vi "Get Properties.vi"(0 "VI Name":string caption="VI Name (\"\")", 5 "AppInst":refnum<vi>, 9 "Scope (0:All)":enum16{"All", "Dynamic"}(ring), 11 "error in":errorcluster) -> (2 "Modifications:VI Modifications Bitset":u64, 3 "File Name Out":string, 4 "Full Name Out":string, 6 "Column Labels":string[](array[string])=["VI Name", "State", "Reentrant", "Reentrancy Type", "FP Behavior", "Code Size", "Data Size", "VI Path"], 8 "Path":path, 10 "Column Data Type":enum16{"String", "Numeric"}[](array[ring]), 12 "ColumnOffsets (Dyn)":i32[](array[numeric])=[1, 1, 1, 5], 13 "VI Properties (Dyn)":string[](array[string]), 14 "VI Properties (All)":string[](array[string]), 15 "error out":errorcluster)   [LabVIEW 2013, in "LVTM.lvlib"]
doc: "Gets the properties at run time of each VI in memory. Set Scope=All to get all properties, set Scope=Dynamic to get only the properties that might change while executing. The later mode will be faster."
uses:
  LVTM.lvlib
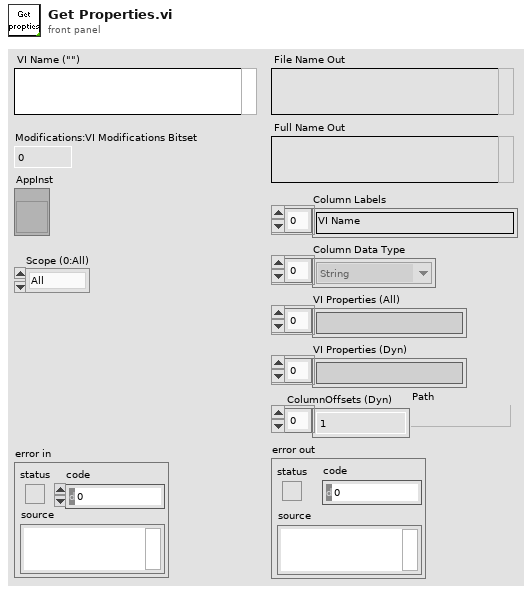
[diagram p1: front panel]
types:
  T1 = enum32{"Bad", "Idle", "Run top level", "Running"}
  T2 = enum16{"Share clones between instances", "Preallocate clone for each instance"}
  T3 = enum32{"Invalid", "Default", "Floating", "Floating/Auto-Hide", "Modal"}
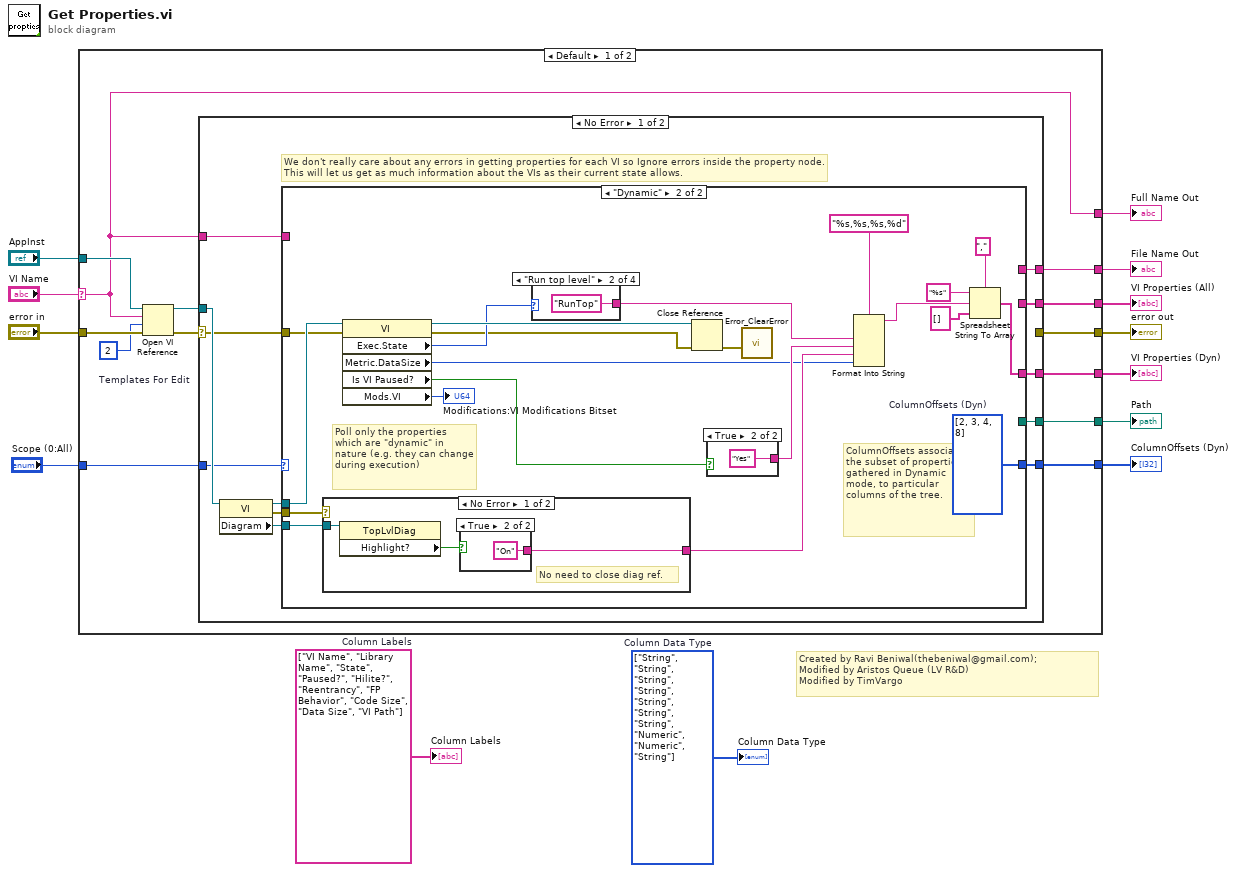
[diagram p0: block diagram]
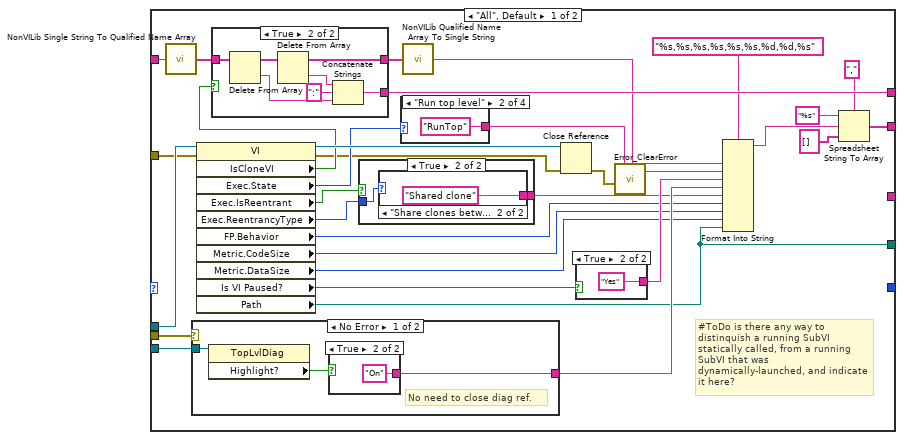
[diagram p2: hidden frame]
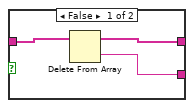
[diagram p3: hidden frame]
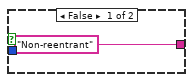
[diagram p4: hidden frame]
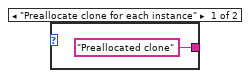
[diagram p5: hidden frame]
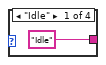
[diagram p6: hidden frame]
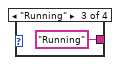
[diagram p7: hidden frame]
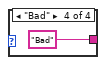
[diagram p8: hidden frame]
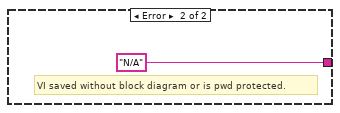
[diagram p10: hidden frame]
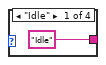
[diagram p12: hidden frame]
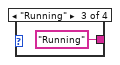
[diagram p13: hidden frame]
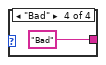
[diagram p14: hidden frame]
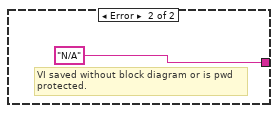
[diagram p16: hidden frame]
diagram:
  w9 = enum16{"String", "Numeric"}[] [enum."String", enum."String", enum."String", enum."String", enum."String", enum."String", enum."String", enum."Numeric", enum."Numeric", enum."String"] items=["String", "Numeric"]  # Column Data Type
  w12 = string[] ["VI Name", "Library Name", "State", "Paused?", "Hilite?", "Reentrancy", "FP Behavior", "Code Size", "Data Size", "VI Path"]  # Column Labels
  # "Created by Ravi Beniwal(thebeniwal@gmail.com);\nModified by Aristos Queue (LV R&D)\nModified by TimVargo"
  n1 = case shown="Default" "VI Name" {
    selector: "VI Name" -> [w20 w128]
    tunnel: [w26 _] -> w13
    tunnel: "error in" -> [w25 w127]
    tunnel: [w20 w128] -> w10
    tunnel: [w22 _] -> w8
    tunnel: "AppInst" -> [w21 _]
    tunnel: [w18 w127] -> w5
    tunnel: "Scope (0:All)" -> [w17 _]
    tunnel: [w16 _] -> w3
    tunnel: [w15 _] -> w2
    tunnel: [w14 _] -> w1
    frame Default {
      w23 = 2  # Templates For Edit
      n2 = Open VI Reference(application reference (local)=w21, vi path=w20, options=w23, error in (no error)=w25) -> (vi reference=w24:refnum<vi>, error out=w19:errorcluster)  [unwired: 2 out]
      n3 = case shown="No Error" w19 {
        selector: w19 -> [w31 w126]
        tunnel: [w38 _] -> w26
        tunnel: w24 -> [w37 _]
        tunnel: [w36 _] -> w22
        tunnel: w20 -> [w35 _]
        tunnel: [_ w126] -> w18
        tunnel: w17 -> [w30 _]
        tunnel: [w29 _] -> w16
        tunnel: [w28 _] -> w15
        tunnel: [w27 _] -> w14
        frame No Error {
          # "We don't really care about any errors in getting properties for each VI so Ignore errors inside the property node.\nThis will let us get as much information about the VIs as their current state allows."
          n4 = property class="VI"(reference=w37) -> (reference out=w33:refnum<vi>, error out=w34:errorcluster, "Diagram"=w32:refnum<vi>)  [unwired: 1 in]
          n5 = case shown="\"Dynamic\"" w30 {
            tunnel: [w69 _] -> w38
            tunnel: [w68 _] -> w36
            tunnel: w35 -> [w67 _]
            tunnel: w34 -> [w56 w108]
            tunnel: w33 -> [w55 w107]
            tunnel: w32 -> [w54 w106]
            tunnel: w31 -> [w43 w100]
            tunnel: [_ w99] -> w29
            tunnel: [_ w98] -> w28
            tunnel: [w39 _] -> w27
            frame "All", Default {
              # "#ToDo is there any way to distinquish a running SubVI statically called, from a running SubVI that was dynamically-launched, and indicate it here?"
              n6 = call "NonVILib Single String To Qualified Name Array.vi"("Fully Qualified String"=w67) -> ("Fully Qualified Array"=w66:string[])
              n7 = case shown="No Error" w56 {
                tunnel: [w89 "N/A"] -> w50
                tunnel: w54 -> [w91 _]
                frame No Error {
                  # "No need to close diag ref."
                  n8 = property class="TopLvlDiag"(reference=w91) -> ("Highlight?"=w90:bool)  [unwired: 1 in, 2 out]
                  n9 = case shown="True" w90 {
                    tunnel: [_ "On"] -> w89
                    frame False {
                    }
                    frame True {
                    }
                  }
                }
                frame Error {
                  # "VI saved without block diagram or is pwd protected."
                }
              }
              n10 = property class="VI"(reference=w55, error in=w43) -> (reference out=w63:refnum<vi>, error out=w42:errorcluster, "IsCloneVI"=w44:bool, "Exec.State"=w53:T1, "Exec.IsReentrant"=w46:bool, "Exec.ReentrancyType"=w40:T2, "FP.Behavior"=w47:T3, "Metric.CodeSize"=w48:u32, "Metric.DataSize"=w49:u32, "Is VI Paused?"=w57:bool, "Path"=w39:path)
              n11 = case shown="True" w44 {
                tunnel: w66 -> [w72 w79]
                tunnel: [w71 w73] -> w68
                tunnel: [w70 w77] -> w65
                frame False {
                  n12 = Delete From Array(array=w72) -> (deleted portion=w71:string, array with subset deleted=w70:string[])  [unwired: 2 in]
                }
                frame True {
                  n13 = Delete From Array(array=w79) -> (deleted portion=w75:string, array with subset deleted=w78:string[])  [unwired: 2 in]
                  n14 = Delete From Array(array=w78) -> (deleted portion=w76:string, array with subset deleted=w77:string[])  [unwired: 2 in]
                  n15 = Concatenate Strings(w76, ":" ("element"), w75) -> (w73:string)
                }
              }
              n16 = case shown="True" w46 {
                tunnel: ["Non-reentrant" w82] -> w45
                tunnel: w40 -> [_ w81]
                frame False {
                }
                frame True {
                  n17 = case shown="\"Share clones between instances\"" w81 {
                    tunnel: ["Preallocated clone" "Shared clone"] -> w82
                    frame "Preallocate clone for each instance" {
                    }
                    frame "Share clones between instances" {
                    }
                  }
                }
              }
              n18 = case shown="\"Run top level\"" w53 {
                tunnel: ["Idle" "RunTop" "Running" "Bad"] -> w52
                frame "Idle" {
                }
                frame "Run top level" {
                }
                frame "Running" {
                }
                frame "Bad" {
                }
              }
              n19 = call "NonVILib Qualified Name Array To Single String.vi"("Fully Qualified Array"=w65) -> ("Fully Qualified String"=w64:string)
              n20 = Close Reference(reference=w63, error in (no error)=w42) -> (error out=w41:errorcluster)
              n21 = case shown="True" w57 {
                tunnel: [_ "Yes"] -> w51
                frame False {
                }
                frame True {
                }
              }
              n22 = call <vilib>:"Error_ClearError.vi"("error in (no error)"=w41) -> ()  [unwired: 10 in, 1 out]
              n23 = Format Into String(format string="%s,%s,%s,%s,%s,%s,%d,%d,%s", w64, w52, w51, w50, w45, w47, w48, w49, w39) -> (resulting string=w58:string)  [unwired: 2 in, 1 out]
              n24 = Spreadsheet String To Array(delimiter (Tab)=",", format string="%s", spreadsheet string=w58, array type (2D Dbl)=string[] [] ("appended array")) -> (array=w69:string[])
            }
            frame "Dynamic" {
              w98 = i32[] [2, 3, 4, 8]  # ColumnOffsets (Dyn)
              # "ColumnOffsets associates the subset of properties, gathered in Dynamic mode, to particular columns of the tree."
              # "Poll only the properties which are \"dynamic\" in nature (e.g. they can change during execution)"
              n25 = case shown="No Error" w108 {
                tunnel: [w120 "N/A"] -> w102
                tunnel: w106 -> [w122 _]
                frame No Error {
                  # "No need to close diag ref."
                  n26 = property class="TopLvlDiag"(reference=w122) -> ("Highlight?"=w121:bool)  [unwired: 1 in, 2 out]
                  n27 = case shown="True" w121 {
                    tunnel: [_ "On"] -> w120
                    frame False {
                    }
                    frame True {
                    }
                  }
                }
                frame Error {
                  # "VI saved without block diagram or is pwd protected."
                }
              }
              n28 = property class="VI"(reference=w107, error in=w100) -> (reference out=w115:refnum<vi>, error out=w97:errorcluster, "Exec.State"=w105:T1, "Metric.DataSize"=w101:u32, "Is VI Paused?"=w109:bool, "Mods.VI"=→"Modifications:VI Modifications Bitset":u64)
              n29 = case shown="\"Run top level\"" w105 {
                tunnel: ["Idle" "RunTop" "Running" "Bad"] -> w104
                frame "Idle" {
                }
                frame "Run top level" {
                }
                frame "Running" {
                }
                frame "Bad" {
                }
              }
              n30 = Close Reference(reference=w115, error in (no error)=w97) -> (error out=w96:errorcluster)
              n31 = case shown="True" w109 {
                tunnel: [_ "Yes"] -> w103
                frame False {
                }
                frame True {
                }
              }
              n32 = call <vilib>:"Error_ClearError.vi"("error in (no error)"=w96) -> ()  [unwired: 10 in, 1 out]
              n33 = Format Into String(format string="%s,%s,%s,%d", w104, w103, w102, w101) -> (resulting string=w110:string)  [unwired: 2 in, 1 out]
              n34 = Spreadsheet String To Array(delimiter (Tab)=",", format string="%s", spreadsheet string=w110, array type (2D Dbl)=string[] [] ("appended array")) -> (array=w99:string[])
            }
          }
        }
        frame Error {
          # "Item is no longer in memory! Pass an error so it will be removed from the Task Manager."
        }
      }
    }
    frame "" {
      # "Adding this blank case let's us use this VI for getting the Col headers. \nIt is just easier to manage the column headers and getting their values in one VI."
    }
  }
  "error out" <- w5
  "VI Properties (All)" <- w13
  "Full Name Out" <- w10
  "File Name Out" <- w8
  "VI Properties (Dyn)" <- w3
  "ColumnOffsets (Dyn)" <- w2
  "Path" <- w1
  "Column Labels" <- w12
  "Column Data Type" <- w9
